vi "XYZStage-Move command (ver 2).vi"(8 "Error In":errorcluster, 9 "XYZ Stage data":T1={"Command"=enum."Initialize", "Channel"="Z", "X"=0.0, "Y"=0.0, "Z"=0.0, "Speed"=0, "Zero"=FALSE, "Use acknowledgement?"=TRUE} {"Speed" format="Speed= %.0f"; "Z" format="Z= %#_g"; "Y" format="Y= %#_g"; "X" format="X= %#_g"}, 11 "XYZ Stage Control in":refnum<class "XYZ Stage Control.lvclass">) -> (0 "Error Out":errorcluster, 1 "Move XYZ command String":string, 3 "XYZ Stage Control out":refnum<class "XYZ Stage Control.lvclass">)   [LabVIEW 2020]
uses:
  Typedefs/XYZ stage data.ctl
  Typedefs/XYZ stage states.ctl
  Typedefs/XYZ channel ring.ctl
  XYZ Stage Control/XYZ Stage Control.lvclass
  XYZ Stage Control/typedefs/XYZ_position_input.ctl
  XYZ Stage Control/typedefs/XYZ axes.ctl
  Typedefs/XYZ_coordinates.ctl
  Typedefs/Command acknowledgment states.ctl
  User Interface/Windows/Position control window/Globals/Pos ctrl window globals.vi
  Globals/gl_XYZStage globals.vi
panel:
  out "Position reached":bool
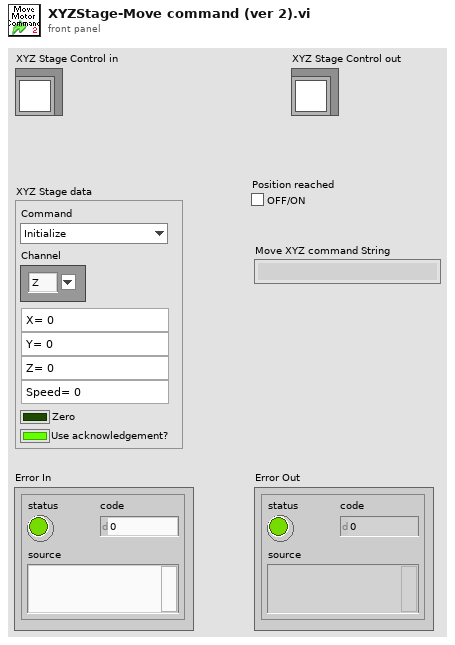
[diagram p1: front panel]
types:
  T1 = typedef "XYZ stage data.ctl" = cluster{"Command":T2, "Channel":T3, "X":sgl, "Y":sgl, "Z":sgl, "Speed":i32, "Zero":bool, "Use acknowledgement?":bool}
  T2 = typedef "XYZ stage states.ctl" = enum16{"Dequeue", "Initialize", "Read Position", "Read Speed Setting", "Move", "Set Max Speed", "Reset Axis", "Stop all movement"}
  T3 = typedef "XYZ channel ring.ctl" = string
  T4 = typedef "XYZ_position_input.ctl" = cluster{"Speed":i32, "Z Limit (um+/-)":sgl, "Axes":T5, "XYZ Coordinates":T6}
  T5 = typedef "XYZ axes.ctl" = string
  T6 = typedef "XYZ_coordinates.ctl" = cluster{"X":sgl, "Y":sgl, "Z":sgl}
  T7 = typedef "Command acknowledgment states.ctl" = enum16{"Acknowledge", "Wait for acknowledgment", "Release queue"}
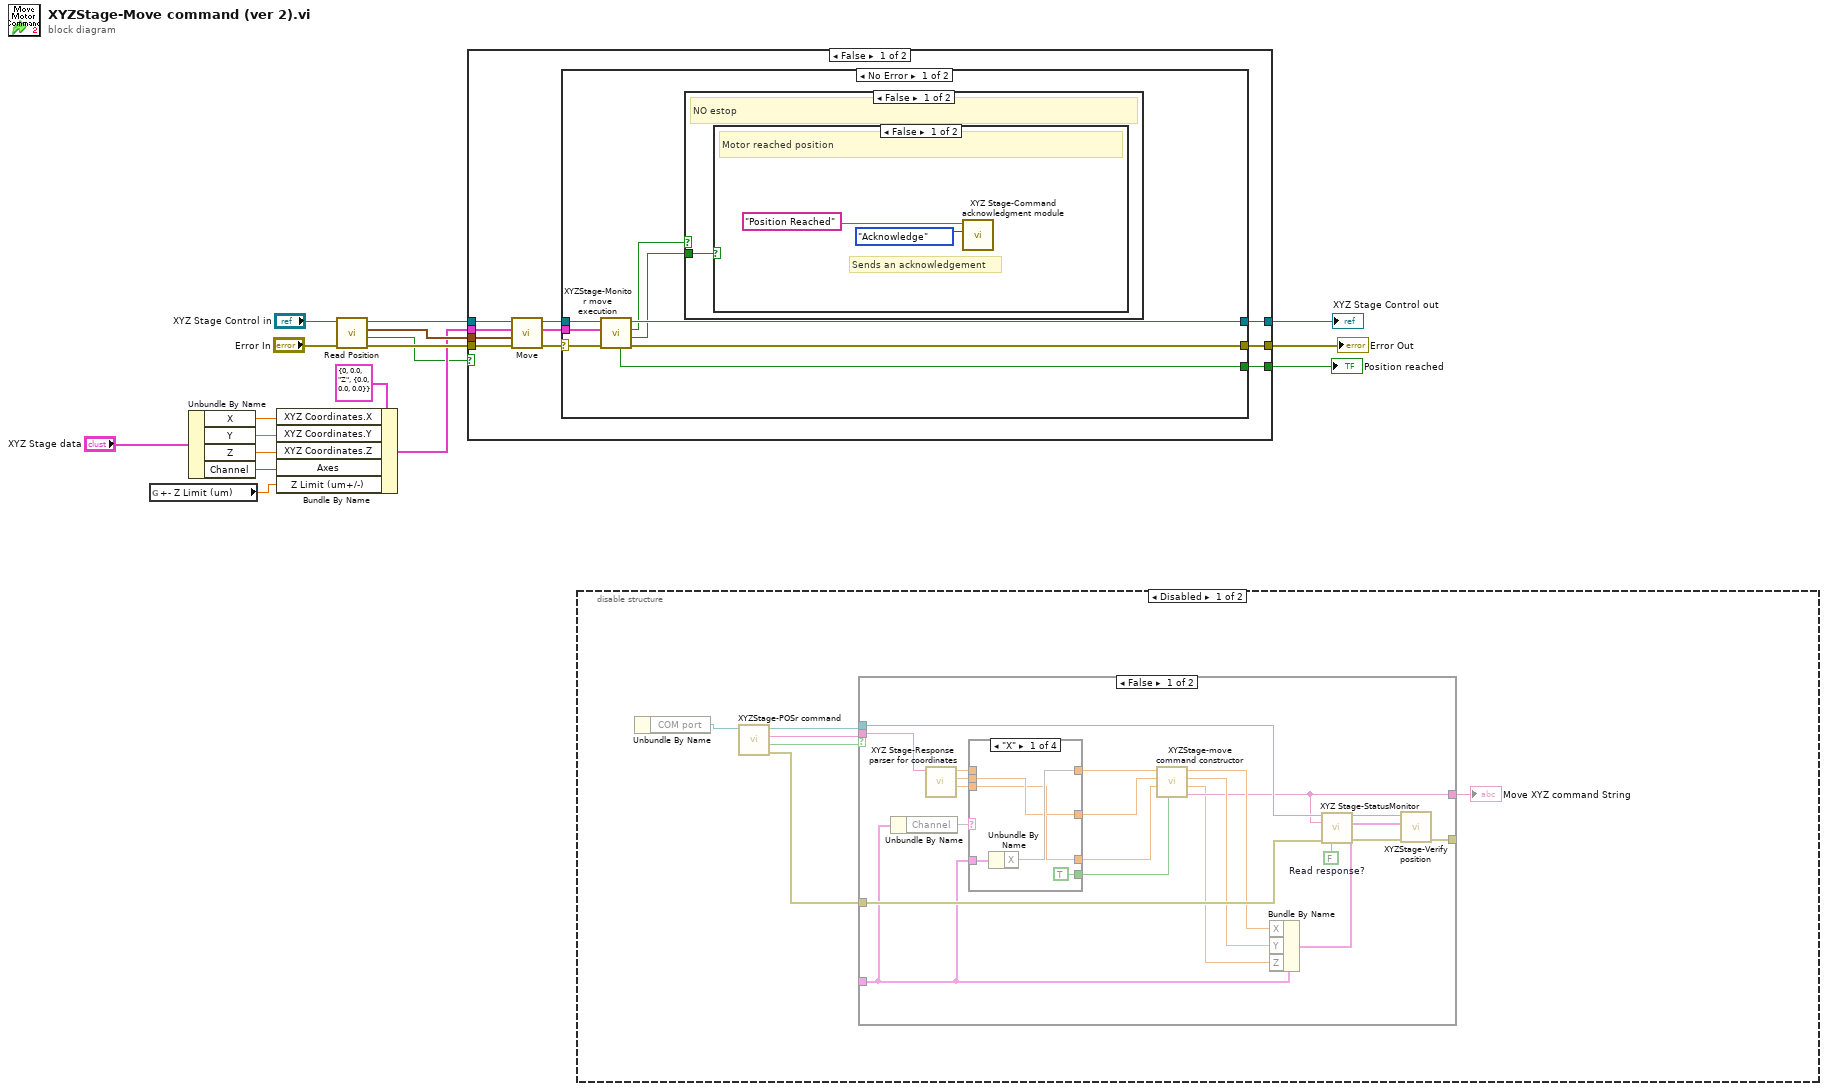
[diagram p0: block diagram]
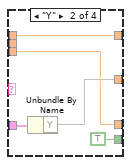
[diagram p2: hidden frame]
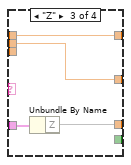
[diagram p3: hidden frame]
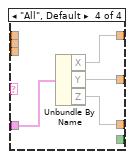
[diagram p4: hidden frame]
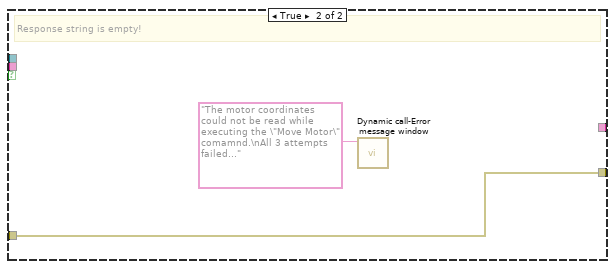
[diagram p5: hidden frame]
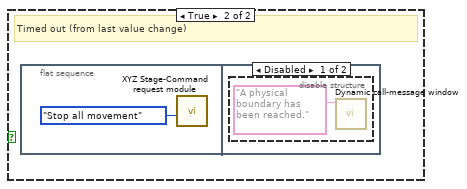
[diagram p7: hidden frame]
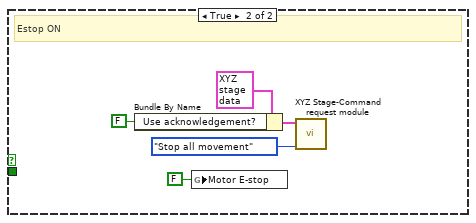
[diagram p9: hidden frame]
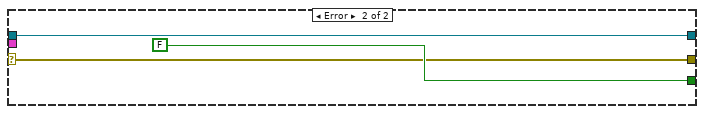
[diagram p10: hidden frame]
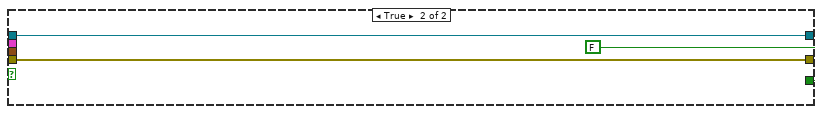
[diagram p11: hidden frame]
diagram:
  n1 = global read "Pos ctrl window globals.vi" "+- Z Limit (um)"() -> (w1:sgl)
  n2 = Unbundle By Name("XYZ Stage data") -> ("X"=w10:sgl, "Y"=w9:sgl, "Z"=w8:sgl, "Channel"=w7:T3)
  n3 = Bundle By Name(cluster=T4 {"Speed"=0, "Z Limit (um+/-)"=0.0, "Axes"="Z", "XYZ Coordinates"={"X"=0.0, "Y"=0.0, "Z"=0.0}} ("XYZ Position Input"), "XYZ Coordinates.X"=w10, "XYZ Coordinates.Y"=w9, "XYZ Coordinates.Z"=w8, "Axes"=w7, "Z Limit (um+/-)"=w1) -> (w6:T4)
  n4 = call-dynamic "Read Position.vi"("error in (no error)"="Error In", "XYZ Stage Control in"="XYZ Stage Control in") -> ("error out"=w14:errorcluster, "No Feedback"=w5:bool, "Stage XYZ Position"=w13:cluster{"X":sgl, "Y":sgl, "Z":sgl}, "XYZ Stage Control out"=w15:refnum<class "XYZ Stage Control.lvclass">)  [unwired: 6 in]
  n5 = case shown="False" w5 {
    tunnel: w15 -> [w27 w51]
    tunnel: w14 -> [w26 w49]
    tunnel: w13 -> [w25 _]
    tunnel: w6 -> [w24 _]
    tunnel: [w21 w51] -> w4
    tunnel: [w20 FALSE ("Position reached")] -> w3
    tunnel: [w18 w49] -> w2
    frame False {
      n6 = call-dynamic "Move.vi"("error in (no error)"=w26, "Current XYZ Position"=w25, "XYZ Position Input"=w24, "XYZ Stage Control in"=w27) -> ("error out"=w19:errorcluster, "XYZ Position Command Output"=w22:T4, "XYZ Stage Control out"=w23:refnum<class "XYZ Stage Control.lvclass">)  [unwired: 5 in]
      n7 = case shown="No Error" w19 {
        selector: w19 -> [w33 w46]
        tunnel: w23 -> [w35 w48]
        tunnel: w22 -> [w28 _]
        tunnel: [w34 w48] -> w21
        tunnel: [w31 FALSE ("Position reached")] -> w20
        tunnel: [w32 w46] -> w18
        frame No Error {
          n8 = call "XYZStage-Monitor move execution.vi"("error in (no error)"=w33, "XYZ Position Command Output"=w28, "XYZ Stage Control in"=w35) -> ("error out"=w32:errorcluster, "Time has Elapsed"=w29:bool, "Motor E-stop"=w30:bool, "XYZ Stage Control out"=w34:refnum<class "XYZ Stage Control.lvclass">, "Position reached"=w31:bool)  [unwired: 4 in]
          n9 = case shown="False" w30 {
            tunnel: w29 -> [w36 _]
            frame False {
              # "NO estop"
              n10 = case shown="False" w36 {
                frame False {
                  # "Sends an acknowledgement"
                  # "Motor reached position"
                  n11 = call "XYZ Stage-Command acknowledgment module.vi"("State"=Command_acknowledgment_states."Acknowledge", "Acknowledgement Message in"="Position Reached") -> ()  [unwired: 7 in, 3 out]
                }
                frame True {
                  # "Timed out (from last value change)"
                  n12 = flat-sequence {
                    frame #0 {
                      n13 = call "XYZ Stage-Command request module.vi"("Command"=XYZ_stage_states."Stop all movement") -> ()  [unwired: 6 in, 5 out]
                    }
                    frame #1 {
                      n14 = disable-structure shown="Disabled" {
                        frame Disabled {
                          n15 = call "Dynamic call-message window.vi"("Message"="A physical boundary has been reached." ("Error Message")) -> ()  [unwired: 10 in, 1 out]
                        }
                        frame Enabled {
                        }
                      }
                    }
                  }
                }
              }
            }
            frame True {
              # "Estop ON"
              n16 = Bundle By Name(cluster=T1 {"Command"=enum."Initialize", "Channel"="Z", "X"=0.0, "Y"=0.0, "Z"=0.0, "Speed"=0, "Zero"=FALSE, "Use acknowledgement?"=TRUE} ("XYZ Stage data to queue"), "Use acknowledgement?"=FALSE) -> (w42:T1)
              n17 = global write "gl_XYZStage globals.vi" "Motor E-stop"(FALSE ("Motor E-stop")) -> ()
              n18 = call "XYZ Stage-Command request module.vi"("Command"=XYZ_stage_states."Stop all movement", "XYZ Stage data to queue"=w42) -> ()  [unwired: 5 in, 5 out]
            }
          }
        }
        frame Error {
        }
      }
    }
    frame True {
    }
  }
  "Error Out" <- w2
  "XYZ Stage Control out" <- w4
  "Position reached" <- w3
  n19 = disable-structure shown="Disabled" {
    frame Disabled {
      n20 = Unbundle By Name() -> ("COM port"=w57:refnum<visa-resource-name>)  [unwired: 1 in]
      n21 = call "XYZStage-POSr command.vi"("VISA Refnum in"=w57) -> ("Error out"=w52:errorcluster, "Empty response string"=w53:bool, "read string"=w56:string, "VISA Refnum out"=w55:refnum<visa-resource-name>)  [unwired: 7 in]
      n22 = case shown="False" w53 {
        tunnel: w52 -> [w79 w99]
        tunnel: w56 -> [w78 _]
        tunnel: w55 -> [w77 _]
        tunnel: [w71 w99] -> w58
        tunnel: _ -> [w67 _]
        tunnel: [w63 _] -> w54
        frame False {
          w69 = FALSE  # Read response?
          n23 = Unbundle By Name(w67) -> ("Channel"=w76)
          n24 = call "XYZ Stage-Response parser for coordinates.vi"("Filtered response string (no CR)"=w78) -> ("Z"=w73:sgl, "Y"=w74:sgl, "X"=w75:sgl)  [unwired: 7 in, 1 out]
          n25 = case shown="\"X\"" w76 {
            tunnel: [w83 w88 w91 w97] -> w62
            tunnel: [w82 w87 w90 w96] -> w68
            tunnel: [w81 w86 w92 w95] -> w61
            tunnel: w67 -> [w84 w89 w93 w94]
            tunnel: w75 -> [_ w88 w91 _]
            tunnel: w74 -> [w82 _ w90 _]
            tunnel: w73 -> [w81 w86 _ _]
            tunnel: [TRUE TRUE _ _] -> w59
            frame "X" {
              n26 = Unbundle By Name(w84) -> ("X"=w83)
            }
            frame "Y" {
              n27 = Unbundle By Name(w89) -> ("Y"=w87)
            }
            frame "Z" {
              n28 = Unbundle By Name(w93) -> ("Z"=w92)
            }
            frame "All", Default {
              n29 = Unbundle By Name(w94) -> ("X"=w97, "Y"=w96, "Z"=w95)
            }
          }
          n30 = call "XYZStage-move command constructor.vi"("Bypass Z-safety interlock"=w59, "Z"=w61, "Y"=w68, "X"=w62) -> ("Move command"=w63:string, "Adjusted Z"=w60:sgl, "Adjusted Y"=w64:sgl, "Adjusted X"=w65:sgl)  [unwired: 3 in, 1 out]
          n31 = Bundle By Name(cluster=w67, "X"=w65, "Y"=w64, "Z"=w60) -> (w66:cluster{})
          n32 = call "XYZ Stage-StatusMonitor.vi"("VISA resource name"=w77, "string to write"=w63, "Error In"=w79, "Read response? (T)"=w69) -> ("VISA resource name out"=w70:refnum<visa-resource-name>, "Error Out"=w72:errorcluster)  [unwired: 7 in, 3 out]
          n33 = call "XYZStage-Verify position.vi"("error in (no error)"=w72, "XYZ Stage data"=w66, "XYZ Stage Port"=w70) -> ("error out"=w71:errorcluster)  [unwired: 8 in]
        }
        frame True {
          # "Response string is empty!"
          n34 = call "Dynamic call-Error message window.vi"("Error Message"="The motor coordinates could not be read while executing the \"Move Motor\" comamnd.\nAll 3 attempts failed...") -> ()  [unwired: 10 in, 1 out]
        }
      }
      "Move XYZ command String" <- w54
    }
    frame Enabled {
    }
  }
